vi "Tokenize String.vi"(8 "error in (no error)":errorcluster, 11 "JSON Lexer in":refnum<class "JSON Lexer.lvclass">) -> (0 "error out":errorcluster, 1 "Tokens":string[](array[string]), 2 "Token Indices":i32[](array[numeric]), 3 "JSON Lexer out":refnum<class "JSON Lexer.lvclass">)   [LabVIEW 2019, in "JKI JSON Serialization.lvlib" / "JSON Lexer.lvclass"]
doc: "JKI Serialization 1.0.0.11\nTomi Maila - JKI\nCopyright (c) 2016, JKI\n\nJKI JSON 1.1.10.37\nTomi Maila - JKI\nCopyright (c) 2017, JKI"
uses:
  JSON Lexer.lvclass
  JSON Lexer.lvclass/JSON Lexer.ctl
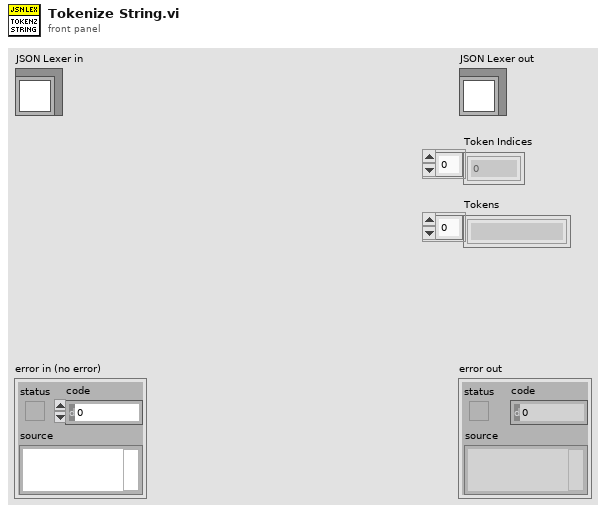
[diagram p1: front panel]
types:
  T1 = typedef "JKI JSON Serialization.lvlib/JSON Lexer.lvclass/JSON Token.ctl" = cluster{"Token Type":T2, "Token Value":string}
  T2 = typedef "JKI JSON Serialization.lvlib/JSON Lexer.lvclass/JSON Token Type.ctl" = enum32{"unknown", "comma", "end-label", "begin-object", "end-object", "begin-array", "end-array", "quoted-string", "boolean", "exponential-number", "decimal-number", "integer-number", "special-number", "null", "symbol", "whitespace", "EOF"}
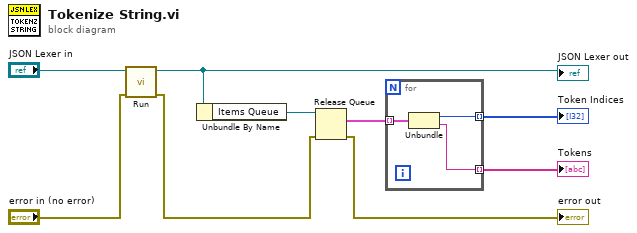
[diagram p0: block diagram]
diagram:
  n1 = call "Run.vi"("error in (no error)"="error in (no error)", "JSON Lexer in"="JSON Lexer in") -> ("error out"=w6:errorcluster, "JSON Lexer out"=w1:refnum<class "JSON Lexer.lvclass">)  [unwired: 8 in]
  "JSON Lexer out" <- w1
  n2 = Unbundle By Name(w1) -> ("Items Queue"=w7:refnum<queue>)
  n3 = Release Queue(queue=w7, error in (no error)=w6) -> (remaining elements=w4:T1[], error out=→"error out":errorcluster)  [unwired: 1 in, 1 out]
  n4 = for {
    tunnel: w4 -> [w12] mode=indexing
    tunnel: [w11] -> w3 mode=indexing
    tunnel: [w10] -> w2 mode=indexing
    n5 = Unbundle(w12) -> ("Token Type"=w11:T2, "Token Value"=w10:string)
  }
  "Token Indices" <- w3
  "Tokens" <- w2
